vi "SimpleGit-LeaveDailyBranch.vi"(11 "path":path) -> (3 "f":string)   [LabVIEW 2017]
uses:
  <vilib>/Hampel Software Engineering/Git API/Git API/GIT-api.lvclass
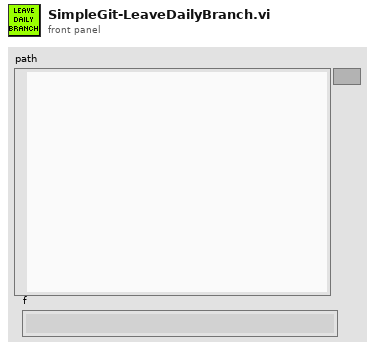
[diagram p1: front panel]
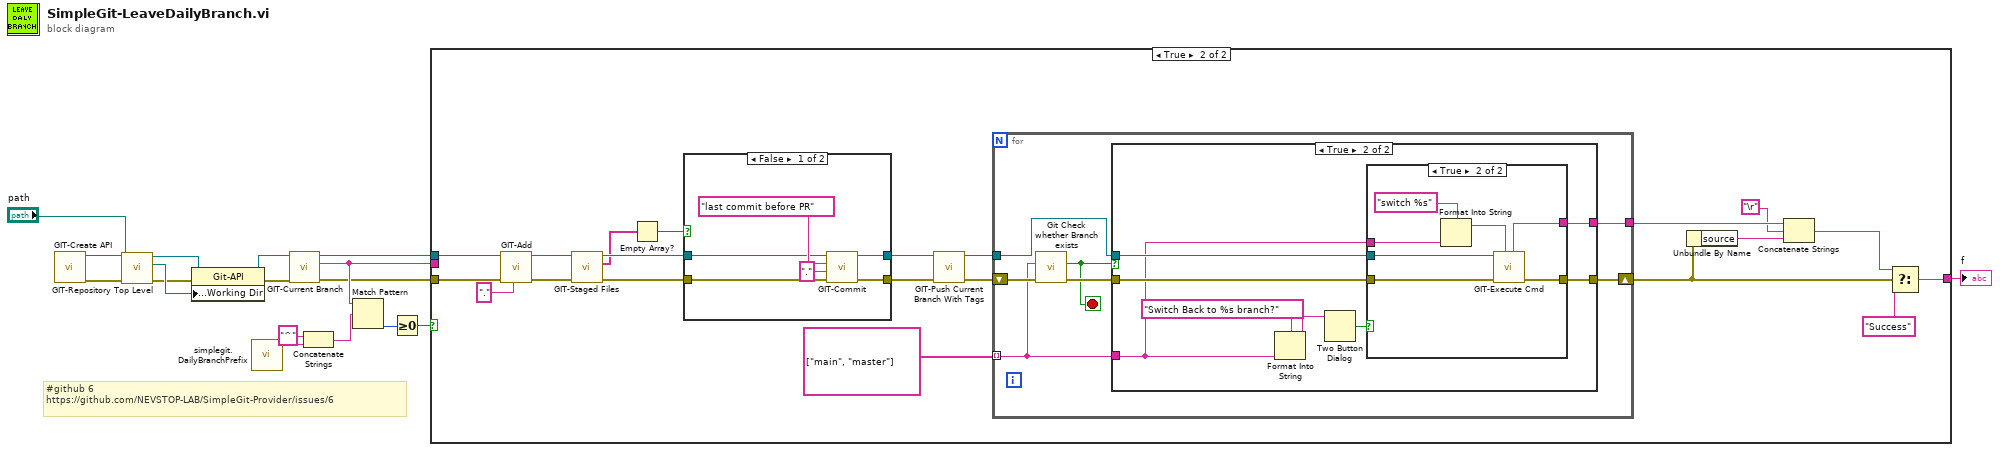
[diagram p0: block diagram]
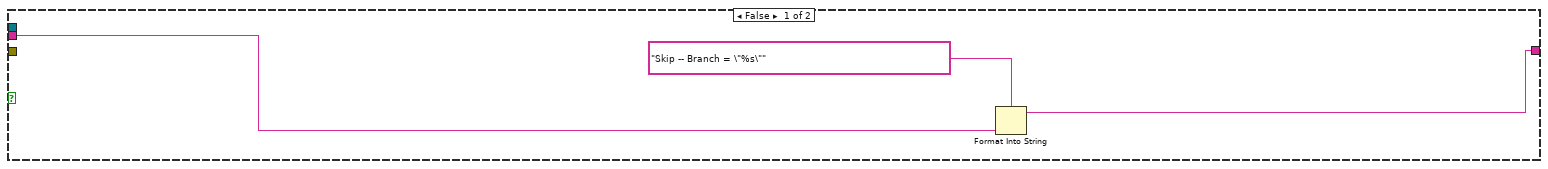
[diagram p2: hidden frame]
diagram:
  # "#github 6\nhttps://github.com/NEVSTOP-LAB/SimpleGit-Provider/issues/6"
  n1 = call <vilib>:"GIT-Create API.vi"() -> ("error out"=w11:errorcluster, "git-api out"=w10:refnum<class "GIT-api.lvclass">)  [unwired: 10 in]
  n2 = call <vilib>:"GIT-Repository Top Level.vi"("error in"=w11, "Current Path"="path", "git-api in"=w10) -> ("error out"=w5:errorcluster, "Repo Top Level Path"=w7:path, "git-api out"=w6:refnum<class "GIT-api.lvclass">)  [unwired: 6 in]
  n3 = property class="Git-API"(reference=w6, error in=w5, "Accessors:Working Dir"=w7) -> (reference out=w8:refnum<class "GIT-api.lvclass">, error out=w9:errorcluster)
  n4 = call "simplegit.DailyBranchPrefix.vi"() -> ("value"=w3:string)  [unwired: 11 in]
  n5 = call <vilib>:"GIT-Current Branch.vi"("error in"=w9, "git-api in"=w8) -> ("error out"=w12:errorcluster, "current branch"=w16:string, "git-api out"=w13:refnum<class "GIT-api.lvclass">)  [unwired: 6 in, 1 out]
  n6 = Concatenate Strings("^" ("string"), w3) -> (w1:string)
  n7 = Match Pattern(string=w16, regular expression=w1) -> (offset past match=w14:i32)  [unwired: 1 in, 3 out]
  n8 = Greater Or Equal To 0?(x=w14) -> (x >= 0?=w15:bool)
  n9 = case shown="True" w15 {
    tunnel: w12 -> [_ w39]
    tunnel: w13 -> [_ w38]
    tunnel: w16 -> [w20 _]
    tunnel: [w18 w24] -> w4
    frame False {
      n10 = Format Into String(format string="Skip -- Branch = \"%s\"" ("f"), w20) -> (resulting string=w18:string)  [unwired: 2 in, 1 out]
    }
    frame True {
      n11 = call <vilib>:"GIT-Add.vi"("param"=".", "error in"=w39, "git-api in"=w38) -> ("error out"=w34:errorcluster, "git-api out"=w36:refnum<class "GIT-api.lvclass">)  [unwired: 6 in, 1 out]
      n12 = call <vilib>:"GIT-Staged Files.vi"("error in"=w34, "Git-API in"=w36) -> ("error out"=w33:errorcluster, "Staged Files"=w32:string[], "Git-API out"=w35:refnum<class "GIT-api.lvclass">)  [unwired: 7 in]
      n13 = Empty Array?(array=w32) -> (empty?=w31:bool)
      n14 = case shown="False" w31 {
        tunnel: [w70 w73] -> w41
        tunnel: [w69 w72] -> w40
        tunnel: w35 -> [w67 w73]
        tunnel: w33 -> [w66 w72]
        frame False {
          n15 = call <vilib>:"GIT-Commit.vi"("error in"=w66, "params"=".", "msg"="last commit before PR", "Git-API in"=w67) -> ("error out"=w69:errorcluster, "Git-API out"=w70:refnum<class "GIT-api.lvclass">)  [unwired: 6 in]
        }
        frame True {
        }
      }
      n16 = call <vilib>:"GIT-Push Current Branch With Tags.vi"("error in"=w40, "Git-API in"=w41) -> ("error out"=w22:errorcluster, "Git-API out"=w23:refnum<class "GIT-api.lvclass">)  [unwired: 8 in]
      n17 = for {
        tunnel: [w48] -> w28
        shift-right: [w47] -> w26
        shift-left: w22 -> [w46]
        tunnel: w23 -> [w42]
        tunnel: string[] ["main", "master"] ("x") -> [w43] mode=indexing
        stop <- w44 stop-if-true
        n18 = call "Git Check whether Branch exists.vi"("error in (no error)"=w46, "DailyPatchBranchName"=w43) -> ("error out"=w45:errorcluster, "Boolean"=w44:bool)  [unwired: 8 in]
        n19 = case shown="True" w44 {
          tunnel: [_ w56] -> w48
          tunnel: [w49 w55] -> w47
          tunnel: w42 -> [_ w54]
          tunnel: w45 -> [w49 w53]
          tunnel: w43 -> [_ w51]
          frame False {
          }
          frame True {
            n20 = Format Into String(format string="Switch Back to %s branch?" ("message"), w51) -> (resulting string=w50:string)  [unwired: 2 in, 1 out]
            n21 = Two Button Dialog(message=w50) -> (T button?=w57:bool)  [unwired: 2 in]
            n22 = case shown="True" w57 {
              tunnel: [w58 w65] -> w55
              tunnel: [_ w64] -> w56
              tunnel: w54 -> [_ w63]
              tunnel: w53 -> [w58 w62]
              tunnel: w51 -> [_ w59]
              frame False {
              }
              frame True {
                n23 = Format Into String(format string="switch %s", w59) -> (resulting string=w60:string)  [unwired: 2 in, 1 out]
                n24 = call <vilib>:"GIT-Execute Cmd.vi"("Command"=w60, "error in"=w62, "Git-API in"=w63) -> ("error out"=w65:errorcluster, "std out"=w64:string)  [unwired: 6 in, 1 out]
              }
            }
          }
        }
      }
      n25 = Unbundle By Name(w26) -> ("source"=w29:string)
      n26 = Concatenate Strings(w28, "\r", w29) -> (w30:string)
      n27 = Select(t=w30, s=w26, f="Success") -> (s? t:f=w24:string)
    }
  }
  "f" <- w4
